vi "FetchRX.vi"(8 "error in (no error)":errorcluster, 11 "reference in":refnum<class "sim_MmW.lvclass">) -> (0 "error out":errorcluster, 2 "RX burst data":refnum<class "mmWave data.lvclass">, 3 "reference out":refnum<class "sim_MmW.lvclass">)   [LabVIEW 2019, in "sim_MmW.lvclass"]
doc: "Fetches RX IQ data from isnturment"
uses:
  sim_MmW.lvclass
  C:/Barkhausen mmWave radar/Development/modules/mmw_instrument/src_LabVIEW/Host/SubVIs/mmWave instrument_class/mmWave instrument.lvclass
  mmWave data_class/mmWave data.lvclass
  mmWave HW Control/HW custom error.ctl
  IQBurst_memo_class/IQBurst_memo.lvclass
  C:/Barkhausen mmWave radar/Development/modules/mmw_instrument/src_LabVIEW/Host/SubVIs/mmWave data_class/mmWave data.lvclass
  mmWave instrument_class/Instrument state.ctl
  mmWave instrument_class/BurstMode.ctl
  d70b2568-79aa-4b08-aecd-bb39ea534b27.vi
  63c303d1-be37-4939-bf5c-023a31352130.vi
  a589e2db-d646-4b58-9dc0-ad384c504dbc.vi
  a53be1d3-6592-4383-ac34-c62b8806fd5b.vi
  032ac389-5447-437e-ad81-02506a350dfa.vi
  87fea010-8960-4ff4-877f-786070fcce39.vi
  <vilib>/Utility/High Resolution Relative Seconds.vi
  <vilib>/Utility/error.llb/Clear Errors.vi
  <vilib>/addons/Modulation/Analog/MT Resample (Complex Cluster).vi
  <vilib>/addons/Modulation/Analog/support/Validators/mod_Fractional Resample Validate.vi
  <vilib>/addons/Modulation/Analog/support/Validators/mod_Check Flush State.vi
  <vilib>/addons/Modulation/Analog/support/mod_FractionalResampler.vi
  <vilib>/addons/Modulation/Analog/support/mod_Integer Rate Interpolation.vi
  <vilib>/addons/Modulation/Analog/support/mod_Set Error Source.vi
  <vilib>/addons/Modulation/Analog/support/Validators/mod_Validate Complex Waveform.vi
  <vilib>/addons/Modulation/Analog/support/mod_PerformResampling.vi
  <vilib>/addons/Modulation/Analog/support/Validators/mod_WFErrorHandler.vi
  <userlib>/_OpenG.lib/string/string.llb/Trim Whitespace (String)__ogtk.vi
  <vilib>/Utility/error.llb/Error Cluster From Error Code.vi
  <vilib>/addons/Modulation/Analog/support/mod_Resampling Factors.vi
  <vilib>/addons/Modulation/Analog/support/mod_ResamplingFilter.vi
  <vilib>/addons/Modulation/Analog/support/mod_Generate Integer Interpolation Filter.vi
  mmWave HW Control/mmWave HW Control.lvlib
  mmWave instrument_class/mmWave instrument.lvclass
  <vilib>/measure/NI_MABase.lvlib
  <vilib>/Analysis/NI_AALBase.lvlib
panel:
  out "final time":dbl format="%#_6p"
  out "elapsed time":dbl format="%#_6p"
  out "size in":i32
  out "size out":i32
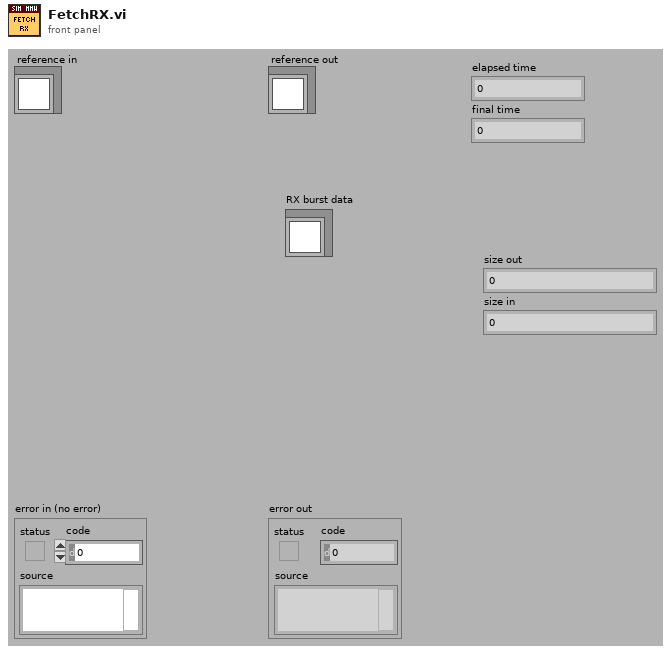
[diagram p1: front panel]
types:
  T1 = typedef "mmWave instrument.lvclass/Instrument state.ctl" = enum16{"Off", "Initialization", "Configuration", "Running", "Calibration"}
  T2 = typedef "mmWave instrument.lvclass/BurstMode.ctl" = enum16{"burst", "continuous"}
  T3 = typedef "mmWave HW Control.lvlib/HW custom error.ctl" = u16
  T4 = typedef "sim_MmW.lvclass/ObjectAttributesRef.ctl" = refnum<data-value>
  T5 = typedef "sim_MmW.lvclass/ObjectAttributes.ctl" = cluster{"RF config":T6, "RX samples":i32, "Downloaded Bursts":map{string, refnum<class "mmWave data.lvclass">}, "TX Fs":dbl, "RX Fs":dbl, "burst sequence":string[], "Burst mode":T2}
  T6 = typedef "mmWave HW Control.lvlib/HW TXRX RF config cluster.ctl" = cluster{"TX.Frequency":dbl, "TX.Gain":dbl, "TX.mmWave adapter":string, "RX.Frequency":dbl, "RX.Gain":dbl, "RX.mmWave adapter":string}
  T7 = typedef "Constants.ctl" = cluster{"data clock rate (Hz)":dbl, "sample rate (Hz)":dbl, "sample rate selector string":string, "default tx bitfile path":path, "default rx bitfile path":path, "default proc bitfile path":path}
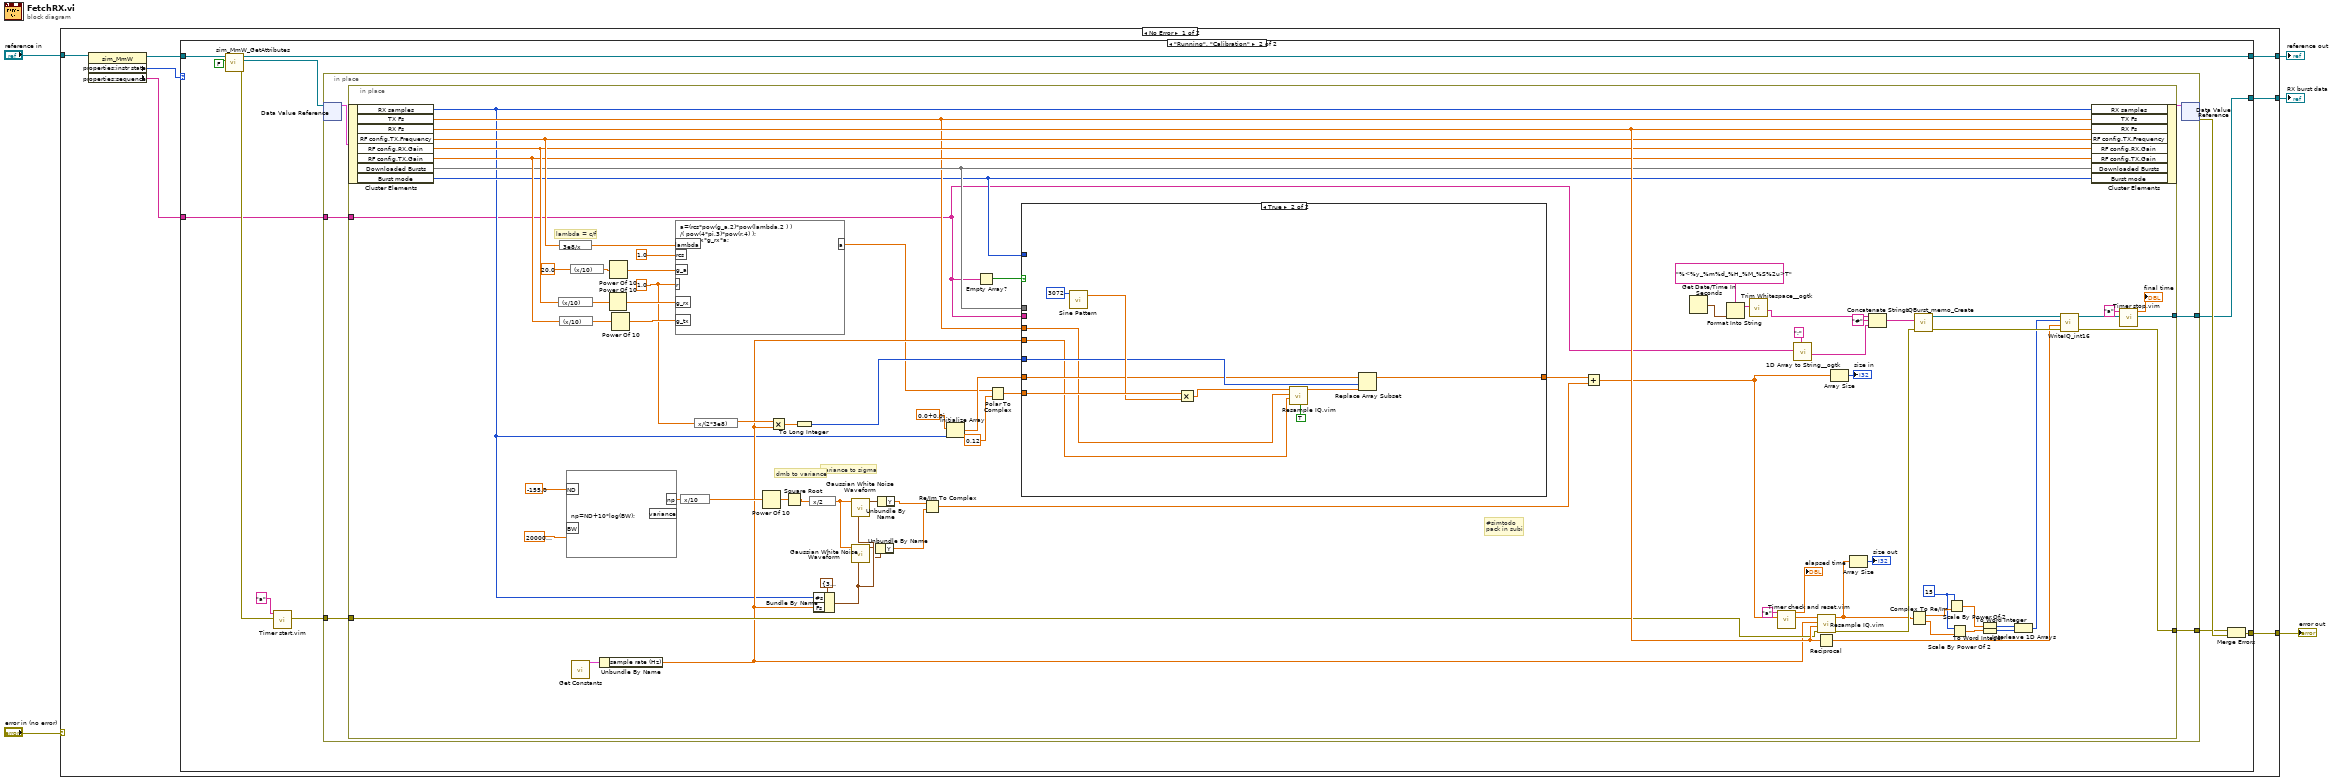
[diagram p0: block diagram]
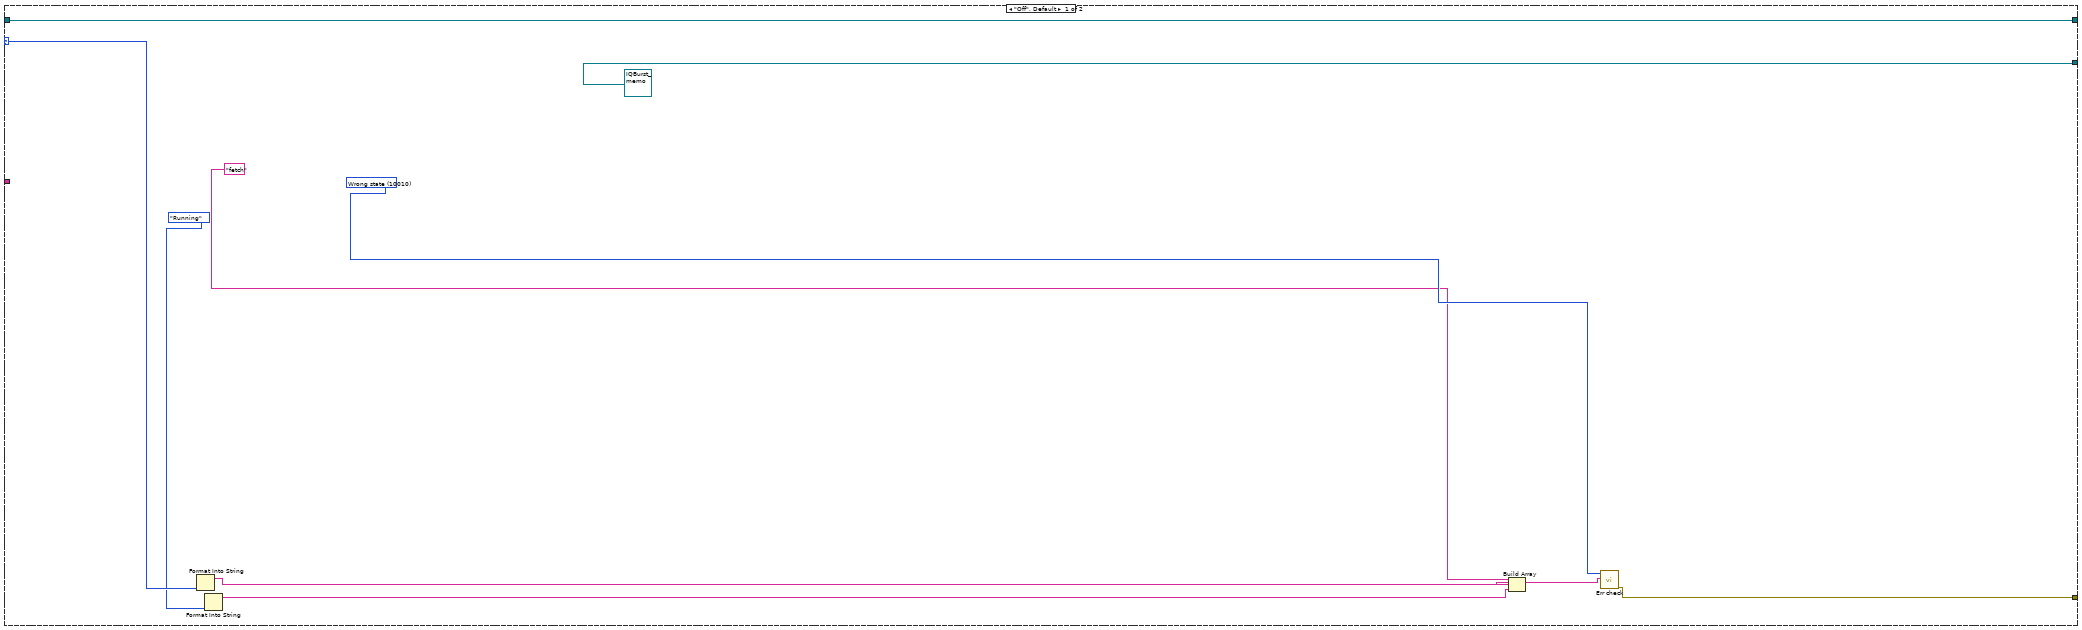
[diagram p2: hidden frame]
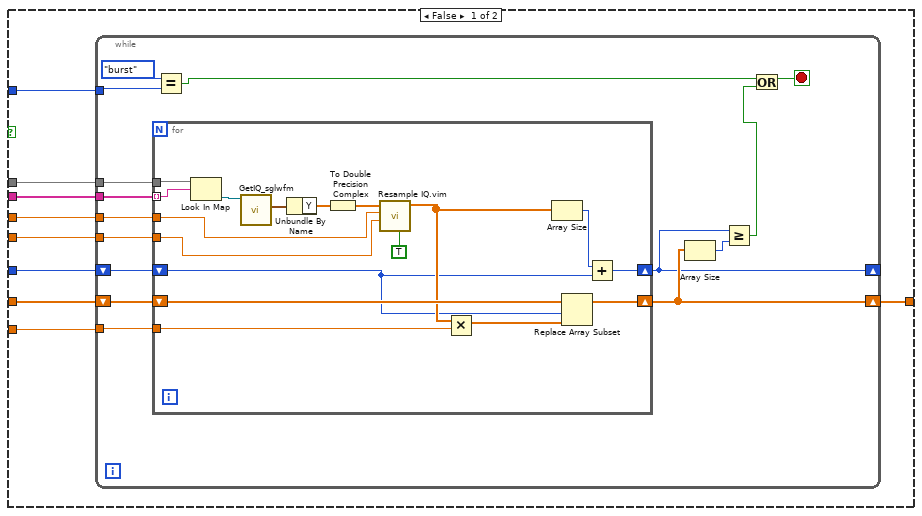
[diagram p3: hidden frame]
diagram:
  n1 = case shown="No Error" "error in (no error)" {
    selector: "error in (no error)" -> [_ w172]
    tunnel: [w12 w172] -> w4
    tunnel: [w11 w171] -> w2
    tunnel: "reference in" -> [w10 w171]
    tunnel: [w7 _] -> w1
    frame No Error {
      n2 = property class="sim_MmW"(reference=w10) -> (reference out=w9:refnum<class "sim_MmW.lvclass">, "properties:instr state"=w8:T1, "properties:sequence"=w6:string[])  [unwired: 1 in, 1 out]
      n3 = case shown="\"Running\", \"Calibration\"" w8 {
        selector: w8 -> [w19 _]
        tunnel: [w16 w34] -> w12
        tunnel: [w22 w31] -> w11
        tunnel: w9 -> [w22 w29]
        tunnel: [refnum<class "IQBurst_memo.lvclass"> refnum ("reference out") w27] -> w7
        tunnel: w6 -> [_ w23]
        frame "Off", Default {
          w21 = T3 10010 items=["TX list"=10000, "TX length"=10001, "RX length"=10002, "Fs"=10003, "RF Fc"=10004, "Wrong state"=10010] ("HW custom err")
          n4 = Format Into String(w19) -> (resulting string=w18:string)  [unwired: 3 in, 1 out]
          n5 = Format Into String(Instrument_state."Running" ("properties:instr state")) -> (resulting string=w13:string)  [unwired: 3 in, 1 out]
          n6 = Build Array("fetch", w18, w13) -> (w17:string[])
          n7 = call "Err check.vi"("Variant Control"=w17, "HW custom err"=w21) -> ("error out"=w16:errorcluster)  [unwired: 9 in]
        }
        frame "Running", "Calibration" {
          n8 = call "sim_MmW_GetAttributes.vi"("return data? (T)"=FALSE, "reference in"=w29) -> ("error out"=w28:errorcluster, "attributes ref"=w30:T4, "reference out"=w31:refnum<class "sim_MmW.lvclass">)  [unwired: 6 in, 1 out]
          n9 = call "Timer start.vim"("dataflow in"=w28, "timer in (t1)"="a") -> ("dataflow out"=w25:errorcluster)  [unwired: 8 in, 1 out]
          n10 = in-place {
            in-place-border: w25 -> [w38]
            in-place-border: [w37] -> w27
            in-place-border: [w36] -> w26
            in-place-border: w23 -> [w35]
            n11 = in-place-dvr #1(w30) -> (w39:T5)  [unwired: 1 out]
            n12 = in-place {
              in-place-border: w38 -> [w103]
              in-place-border: [w60] -> w37
              in-place-border: [w106] -> w36
              in-place-border: w35 -> [w41]
              w49 = i16 15 ("n")
              w86 = 1.0 ("input variable")
              # "variance to sigma"
              # "dmb to variance"
              # "lambda = c/f"
              # "#simtodo\npack in subi"
              n13 = in-place-cluster #2(w39) -> ("RX samples"=w73:i32, "TX Fs"=w80:dbl, "RX Fs"=w108:dbl, "RF config.TX.Frequency"=w102:dbl, "RF config.RX.Gain"=w98:dbl, "RF config.TX.Gain"=w95:dbl, "Downloaded Bursts"=w82:map{string, refnum<class "mmWave data.lvclass">}, "Burst mode"=w76:T2)
              n14 = expression code="(x/10)"(w98) -> (w97:dbl)
              n15 = expression code="3e8/x"(w102) -> (w101:dbl)
              n16 = expression code="(x/10)"(w95) -> (w96:dbl)
              n17 = formula code="np=ND+10*log(BW);"("ND"=-155.0 ("Noise density"), "BW"=2000000000.0) -> ("np"=w88:dbl)  [unwired: 1 out]
              n18 = expression code="(x/10)"(20.0 ("input variable")) -> (w94:dbl)
              n19 = call "Get Constants.vi"() -> ("constants"=w115:T7)  [unwired: 15 in]
              n20 = Unbundle By Name(w115) -> ("sample rate (Hz)"=w81:dbl)
              n21 = Power Of 10(x=w97) -> (10^x=w91:dbl)
              n22 = Power Of 10(x=w94) -> (10^x=w93:dbl)
              n23 = Power Of 10(x=w96) -> (10^x=w92:dbl)
              n24 = formula code="a=(rcs*pow(g_a,2)*pow(lambda,2 ) )\n/( pow(4*pi,3)*pow(r,4) );\na= g_tx*g_rx*a;"("lambda"=w101, "rcs"=1.0 ("input variable"), "g_a"=w93, "r"=w86, "g_rx"=w91, "g_tx"=w92) -> ("a"=w47:dbl)
              n25 = expression code="x/10"(w88) -> (w87:dbl)
              n26 = expression code="x/(2*3e8)"(w86) -> (w85:dbl)
              n27 = Power Of 10(x=w87) -> (10^x=w72:dbl)
              n28 = Multiply(x=w85, y=w81) -> (x*y=w84:dbl)
              n29 = Square Root(x=w72) -> (sqrt(x)=w71:dbl)
              n30 = To Long Integer(number=w84) -> (32bit integer=w83:i32)
              n31 = expression code="x/2"(w71) -> (w64:dbl)
              n32 = Bundle By Name(cluster=cluster{"Fs":dbl, "#s":dbl} {"Fs"=3072000000.0, "#s"=16000.0} ("sampling info"), "#s"=w73, "Fs"=w81) -> (w69:cluster{"Fs":dbl, "#s":dbl})
              n33 = call <vilib>:"Gaussian White Noise Waveform.vi"("sampling info"=w69, "standard deviation"=w64) -> ("signal out"=w68:waveform(dbl))  [unwired: 8 in, 1 out]
              n34 = call <vilib>:"Gaussian White Noise Waveform.vi"("sampling info"=w69, "standard deviation"=w64) -> ("signal out"=w67:waveform(dbl))  [unwired: 8 in, 1 out]
              n35 = Unbundle By Name(w67) -> ("Y"=w66:dbl[])
              n36 = Unbundle By Name(w68) -> ("Y"=w65:dbl[])
              n37 = Re/Im To Complex(1:w66, 2:w65) -> (0:w77:cdb[])
              n38 = Initialize Array(cdb 0.0+0.0i, w73) -> (w79:cdb[])
              n39 = Empty Array?(array=w41) -> (empty?=w44:bool)
              n40 = Polar To Complex(1:0.12 ("theta"), 2:w47) -> (0:w45:cdb)
              n41 = case shown="True" w44 {
                tunnel: w83 -> [w127 w167]
                tunnel: w82 -> [w126 _]
                tunnel: w81 -> [w125 w161]
                tunnel: w80 -> [w124 w160]
                tunnel: w79 -> [w123 w166]
                tunnel: w76 -> [w122 _]
                tunnel: [w121 w165] -> w75
                tunnel: w45 -> [w120 w169]
                tunnel: w41 -> [w119 _]
                frame False {
                  n42 = while {
                    tunnel: w126 -> [w141]
                    tunnel: w119 -> [w140]
                    tunnel: w125 -> [w139]
                    tunnel: w124 -> [w138]
                    tunnel: w120 -> [w136]
                    shift-right: [w131] -> w121
                    shift-left: w123 -> [w137]
                    tunnel: w122 -> [w135]
                    shift-right: [w128] -> _
                    shift-left: w127 -> [w142]
                    stop <- w129 stop-if-true
                    n43 = for {
                      shift-right: [w147] -> w128
                      shift-left: w142 -> [w146]
                      shift-right: [w152] -> w131
                      shift-left: w137 -> [w153]
                      tunnel: w141 -> [w159]
                      tunnel: w140 -> [w158] mode=indexing
                      tunnel: w139 -> [w148]
                      tunnel: w138 -> [w149]
                      tunnel: w136 -> [w143]
                      n44 = Look In Map(map=w159, key=w158) -> (value=w157:refnum<class "mmWave data.lvclass">)  [unwired: 1 in, 1 out]
                      n45 = call-dynamic "GetIQ_sglwfm.vi"("reference in"=w157) -> ("IQ"=w156:waveform(csg))  [unwired: 8 in, 2 out]
                      n46 = Unbundle By Name(w156) -> ("Y"=w155:csg[])
                      n47 = To Double Precision Complex(1:w155) -> (0:w154:cdb[])
                      n48 = call "Resample IQ.vim"("flush buffers? (T"=TRUE ("flush buffers? (F)"), "FS out"=w148, "Fs in"=w149, "data in"=w154) -> ("resampled data"=w150:cdb[])  [unwired: 6 in, 1 out]
                      n49 = Multiply(x=w150, y=w143) -> (x*y=w144:cdb[])
                      n50 = Array Size(array=w150) -> (size(s)=w145:i32)
                      n51 = Replace Array Subset(array=w153, new element=w144, index=w146) -> (w152:cdb[])
                      n52 = Add(x=w145, y=w146) -> (x+y=w147:i32)
                    }
                    n53 = Equal?(x=BurstMode."burst", y=w135) -> (x = y?=w133:bool)
                    n54 = Array Size(array=w131) -> (size(s)=w132:i32)
                    n55 = Greater Or Equal?(x=w128, y=w132) -> (x >= y?=w130:bool)
                    n56 = Or(x=w133, y=w130) -> (x .or. y?=w129:bool)
                  }
                }
                frame True {
                  n57 = call <vilib>:"Sine Pattern.vi"("samples"=3072) -> ("Sinusoidal Pattern"=w168:dbl[])  [unwired: 3 in, 1 out]
                  n58 = Multiply(x=w169, y=w168) -> (x*y=w163:cdb[])
                  n59 = call "Resample IQ.vim"("flush buffers? (T"=TRUE ("flush buffers? (F)"), "FS out"=w161, "Fs in"=w160, "data in"=w163) -> ("resampled data"=w162:cdb[])  [unwired: 6 in, 1 out]
                  n60 = Replace Array Subset(array=w166, new element=w162, index=w167) -> (w165:cdb[])
                }
              }
              n61 = Add(x=w75, y=w77) -> (x+y=w78:cdb[])
              n62 = Get Date/Time In Seconds() -> (seconds since 1Jan1904=w118:timestamp)
              n63 = Format Into String(format string="%<%y_%m%d_%H_%M_%S%2u>T", w118) -> (resulting string=w116:string)  [unwired: 2 in, 1 out]
              n64 = call-poly <userlib>:"Trim Whitespace__ogtk.vi"("String in"=w116) -> ("String out"=w114:string)  [unwired: 6 in]
              n65 = call "Timer check and reset.vim"("dataflow in"=w78, "timer name (t1)"="a") -> ("dataflow out"=w63:cdb[], "elapsed time"=→"elapsed time":dbl)  [unwired: 8 in]
              n66 = call <userlib>:"1D Array to String__ogtk.vi"("delimiter (Tab)"=";", "Array of Strings"=w41) -> ("delimited string"=w42:string)  [unwired: 9 in]
              n67 = Reciprocal(x=w108) -> (1/x=w48:dbl)
              n68 = call "Resample IQ.vim"("error in (no error)"=w103, "FS out"=w108, "Fs in"=w81, "data in"=w63) -> ("error out"=w107:errorcluster, "resampled data"=w51:cdb[])  [unwired: 6 in]
              n69 = Array Size(array=w78) -> (size(s)=→"size in":i32)
              n70 = Array Size(array=w51) -> (size(s)=→"size out":i32)
              n71 = Concatenate Strings(w114, "#" ("string"), w42) -> (w112:string)
              n72 = Complex To Re/Im(x + iy=w51) -> (x=w57:dbl[], y=w56:dbl[])
              n73 = call "IQBurst_memo_Create.vi"("error in (no error)"=w107, "burst name"=w112) -> ("error out"=w111:errorcluster, "reference out"=w110:refnum<class "IQBurst_memo.lvclass">)  [unwired: 8 in]
              n74 = Scale By Power Of 2(n=w49, x=w57) -> (x*2^n=w54:dbl[])
              n75 = Scale By Power Of 2(n=w49, x=w56) -> (x*2^n=w55:dbl[])
              n76 = To Word Integer(number=w54) -> (16bit integer=w53:i16[])
              n77 = To Word Integer(number=w55) -> (16bit integer=w52:i16[])
              n78 = Interleave 1D Arrays(w53, w52) -> (w50:i16[])
              n79 = call-dynamic "WriteIQ_int16.vi"("error in (no error)"=w111, "dt"=w48, "data"=w50, "reference in"=w110) -> ("error out"=w106:errorcluster, "reference out"=w109:refnum<class "IQBurst_memo.lvclass">)  [unwired: 6 in]
              n80 = in-place-cluster #2("RX samples"=w73, "TX Fs"=w80, "RX Fs"=w108, "RF config.TX.Frequency"=w102, "RF config.RX.Gain"=w98, "RF config.TX.Gain"=w95, "Downloaded Bursts"=w82, "Burst mode"=w76) -> (w40:T5)
              n81 = call "Timer stop.vim"("dataflow in"=w109, "timer name (t1)"="a") -> ("dataflow out"=w60:refnum<class "IQBurst_memo.lvclass">, "final time"=→"final time":dbl)  [unwired: 8 in]
            }
            n82 = in-place-dvr #1(w40) -> (w33:errorcluster)  [unwired: 1 out]
          }
          n83 = Merge Errors(w26, w33) -> (w34:errorcluster)
        }
      }
    }
    frame Error {
    }
  }
  "error out" <- w4
  "reference out" <- w2
  "RX burst data" <- w1
